vi "PH_OceanOpticsSpectrometer.set Failure.vi"(0 "i ref in":refnum<vi>, 5 "error IO":errorcluster) -> (14 "i ref out":refnum<vi>, 19 "error out":errorcluster)   [LabVIEW 2014, in "PH_OceanOpticsSpectrometer.lvlib"]
doc: "This VI sets related GUI elements and the statues service to failure mode."
uses:
  PH_OceanOpticsSpectrometer.lvlib
  PH_Basics/PH_StatusHandler/PH_StatusHandler.Status.ctl
  PH_OceanOpticsSpectrometer.Trigger.ctl
  PH_Basics/PH_StatusHandler/PH_StatusHandler.lvlib
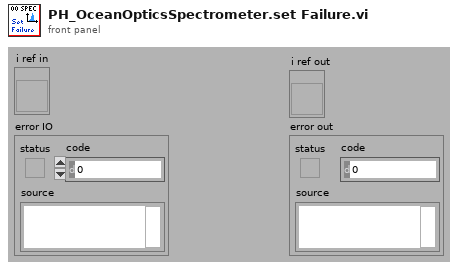
[diagram p1: front panel]
types:
  T1 = typedef "PH_OceanOpticsSpectrometer.lvlib/PH_OceanOpticsSpectrometer.i attribute.ctl" = cluster{"GUI Refs":cluster{"Delete":refnum<vi>, "Spectrum":refnum<vi>, "Display Width":refnum<vi>, "Display Center":refnum<vi>, "Save":refnum<vi>, "Integration time":refnum<vi>, "center wavelength":refnum<vi>, "width":refnum<vi>, "Wanted Trigger Mode":refnum<vi>, "Current Trigger Mode":refnum<vi>, "Trigger Info":refnum<vi>, "Model":refnum<vi>, "Driver":refnum<vi>, "Firmware":refnum<vi>}, "Display":cluster{"Width":dbl, "Center":dbl}, "VISA resource name":refnum<visa-resource-name>, "Integration time [ms]":cluster{"Current Value":u16, "Wanted Value":u16}, "Trigger":cluster{"Current value":T2, "Wanted value":T2}, "Default VISA Timeout":u32, "Last Data":cluster{"Wavelength Bins":dbl[], "Spectrum by Pixels":dbl[]}}
  T2 = typedef "PH_OceanOpticsSpectrometer.lvlib/PH_OceanOpticsSpectrometer.Trigger.ctl" = enum32{"External", "Normal"}
  T3 = typedef "PH_StatusHandler.lvlib/PH_StatusHandler.Status.ctl" = i16
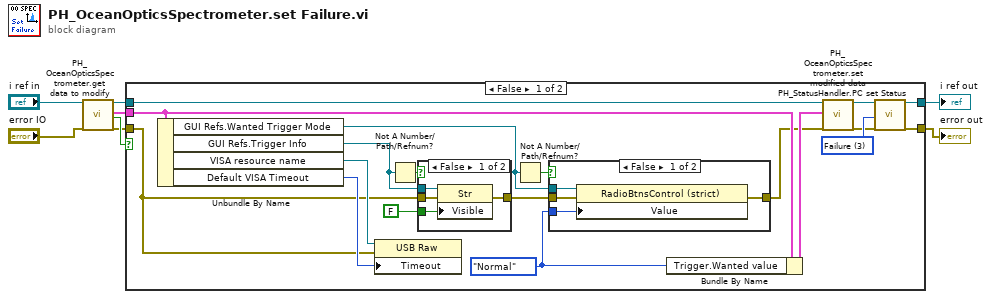
[diagram p0: block diagram]
diagram:
  n1 = call "PH_OceanOpticsSpectrometer.get data to modify.vi"("i ref in"="i ref in", "error in (no error)"="error IO") -> ("i ref out"=w2:refnum<vi>, "i attribute"=w4:T1, "timed out"=w3:bool, "error out"=w1:errorcluster)  [unwired: 14 in]
  n2 = case shown="False" w3 {
    tunnel: w1 -> [w18 w38]
    tunnel: [w9 w38] -> w7
    tunnel: w2 -> [w27 w39]
    tunnel: [w11 w39] -> w6
    tunnel: w4 -> [w25 _]
    frame False {
      w21 = PH_OceanOpticsSpectrometer.Trigger."Normal" ("Trigger.Wanted value")
      w24 = T3 3 items=["no info", "off/false/out", "on/true/in", "Failure", "Alarm", "Status 1", "Status 2", "Status 3"] ("Device Status")
      n3 = Unbundle By Name(w25) -> ("GUI Refs.Wanted Trigger Mode"=w22:refnum<vi>, "GUI Refs.Trigger Info"=w15:refnum<vi>, "VISA resource name"=w20:refnum<visa-resource-name>, "Default VISA Timeout"=w19:u32)
      n4 = property class="USB Raw"(reference=w20, error in=w18, "Timeout"=w19) -> ()  [unwired: 2 out]
      n5 = Not A Number/Path/Refnum?(number/path/refnum=w15) -> (NaN/Path/Refnum?=w16:bool)
      n6 = case shown="False" w16 {
        tunnel: w15 -> [w30 _]
        tunnel: w18 -> [w31 w32]
        tunnel: [w29 w32] -> w17
        tunnel: FALSE ("Visible") -> [w28 _]
        frame False {
          n7 = property class="Str"(reference=w30, error in=w31, "Visible"=w28) -> (error out=w29:errorcluster)  [unwired: 1 out]
        }
        frame True {
        }
      }
      n8 = Not A Number/Path/Refnum?(number/path/refnum=w22) -> (NaN/Path/Refnum?=w23:bool)
      n9 = case shown="False" w23 {
        tunnel: w22 -> [w35 _]
        tunnel: w17 -> [w36 w37]
        tunnel: [w34 w37] -> w13
        tunnel: w21 -> [w33 _]
        frame False {
          n10 = property class="RadioBtnsControl (strict)"(reference=w35, error in=w36, "Value"=w33) -> (error out=w34:errorcluster)  [unwired: 1 out]
        }
        frame True {
        }
      }
      n11 = Bundle By Name(cluster=w25, "Trigger.Wanted value"=w21) -> (w26:T1)
      n12 = call "PH_OceanOpticsSpectrometer.set modified data.vi"("i ref in"=w27, "i attribute"=w26, "error in (no error)"=w13) -> ("i ref out"=w12:refnum<vi>, "error out"=w10:errorcluster)  [unwired: 15 in]
      n13 = call "PH_StatusHandler.PC set Status.vi"("i ref in"=w12, "Status"=w24, "error in (no error)"=w10) -> ("i ref out"=w11:refnum<vi>, "error out"=w9:errorcluster)  [unwired: 15 in]
    }
    frame True {
    }
  }
  "error out" <- w7
  "i ref out" <- w6
